vi "Conver.vi"() -> ()   [LabVIEW 2021]
panel:
  out "0, 1":i16
  out "String 5":string
  out "Boolean 5":bool
  out "Numeric 10":dbl
  out "Numeric 9":u8
  out "String 4":string
  out "Boolean 4":bool
  out "Numeric 8":dbl
  out "Numeric 7":u8
  out "String 3":string
  out "Boolean 3":bool
  out "Numeric 6":dbl
  out "Numeric 3":u8
  out "Numeric 5":dbl
  out "Boolean 2":bool
  out "String 2":string
  in  "String":string
  in  "Boolean":bool
  in  "Numeric 2":u8
  in  "Numeric":dbl
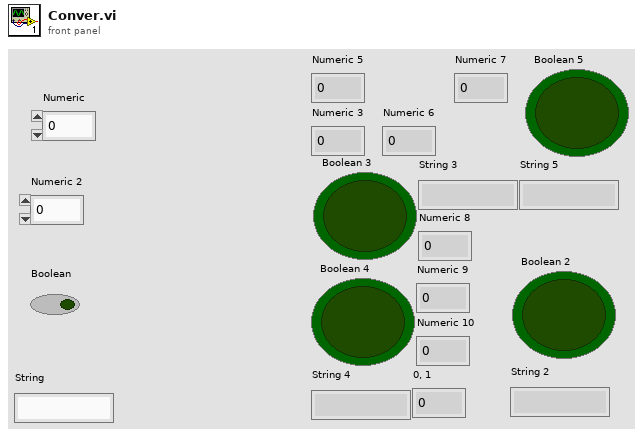
[diagram p1: front panel]
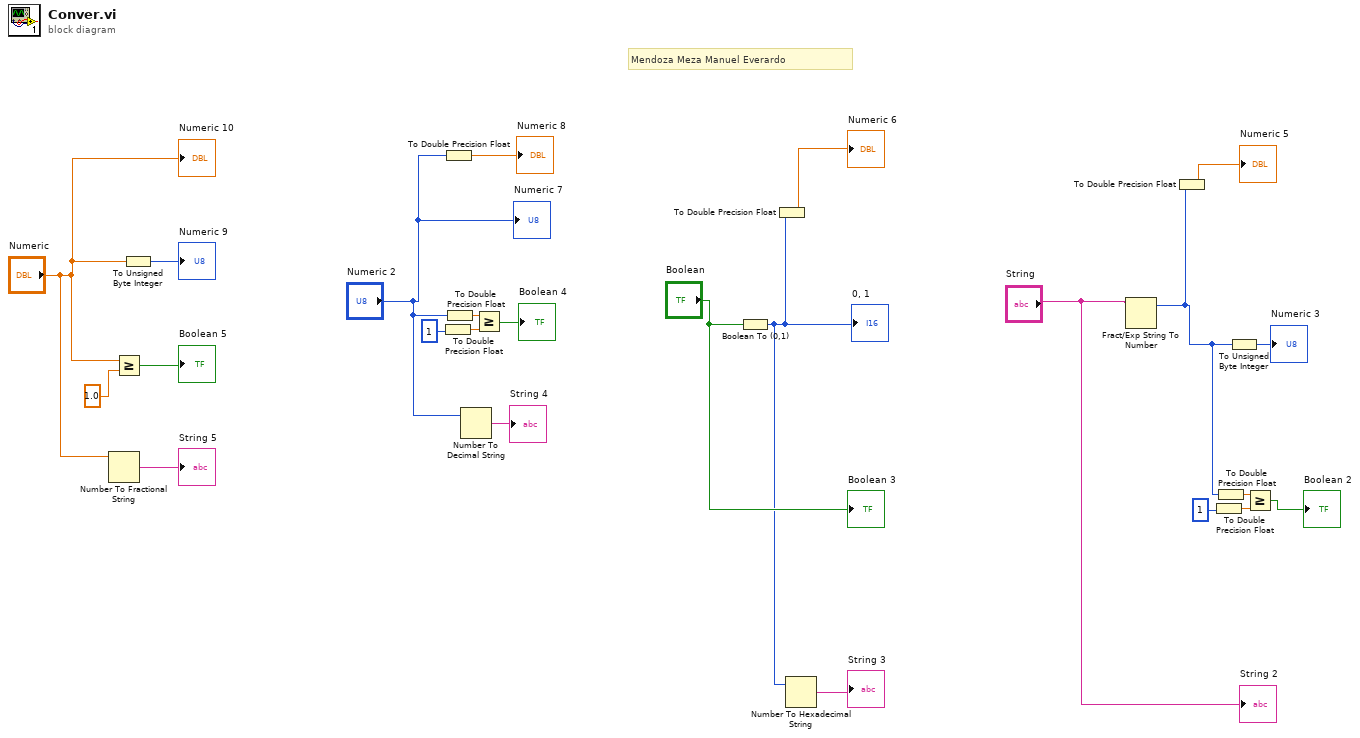
[diagram p0: block diagram]
diagram:
  # "Mendoza Meza Manuel Everardo"
  n1 = Number To Fractional String(number="Numeric") -> (F-format string=→"String 5":string)  [unwired: 3 in]
  n2 = Greater Or Equal?(x="Numeric", y=1.0) -> (x >= y?=→"Boolean 5":bool)
  n3 = To Unsigned Byte Integer(number="Numeric") -> (unsigned 8bit integer=→"Numeric 9":u8)
  n4 = To Double Precision Float(number=1) -> (double precision float=w10:dbl)
  n5 = To Double Precision Float(number="Numeric 2") -> (double precision float=→"Numeric 8":dbl)
  n6 = To Double Precision Float(number="Numeric 2") -> (double precision float=w11:dbl)
  n7 = Number To Decimal String(number="Numeric 2") -> (decimal integer string=→"String 4":string)  [unwired: 1 in]
  n8 = Greater Or Equal?(x=w11, y=w10) -> (x >= y?=→"Boolean 4":bool)
  n9 = Boolean To (0,1)(Boolean="Boolean") -> (0, 1=w19:i16)
  "0, 1" <- w19
  n10 = To Double Precision Float(number=w19) -> (double precision float=→"Numeric 6":dbl)
  n11 = Number To Hexadecimal String(2:w19) -> (0:→"String 3":string)  [unwired: 1 in]
  n12 = Fract/Exp String To Number(string="String") -> (offset past number=w3:i32)  [unwired: 3 in, 1 out]
  n13 = To Double Precision Float(number=w3) -> (double precision float=→"Numeric 5":dbl)
  n14 = To Double Precision Float(number=1) -> (double precision float=w6:dbl)
  n15 = To Double Precision Float(number=w3) -> (double precision float=w5:dbl)
  n16 = To Unsigned Byte Integer(number=w3) -> (unsigned 8bit integer=→"Numeric 3":u8)
  n17 = Greater Or Equal?(x=w5, y=w6) -> (x >= y?=→"Boolean 2":bool)
  "String 2" <- "String"
  "Boolean 3" <- "Boolean"
  "Numeric 7" <- "Numeric 2"
  "Numeric 10" <- "Numeric"
